vi "Z stage safety.vi"(7 "new position":dbl format="%#_13g", 8 "Error In":errorcluster, 10 "Table Stages":T1={"X Stage"={"Position"=0.0, "Is.Enabled?"=FALSE, "Is.Connected?"=FALSE, "Device SN"="45876539", "AccelerationMaximum"=0.0, "VelocityMaximum"=0.0, "Acceleration"=0.0, "Velocity"=0.0, "waitTimeout (ms)"=0, "Model"=enum."None", "Is.Homed?"=FALSE, "MOVE"=FALSE}, "Y Stage"={"Position"=0.0, "Is.Enabled?"=FALSE, "Is.Connected?"=FALSE, "Device SN"="45876539", "AccelerationMaximum"=0.0, "VelocityMaximum"=0.0, "Acceleration"=0.0, "Velocity"=0.0, "waitTimeout (ms)"=0, "Model"=enum."None", "Is.Homed?"=FALSE, "MOVE"=FALSE}, "Z Stage"={"Position"=0.0, "Is.Enabled?"=FALSE, "Is.Connected?"=FALSE, "Device SN"="45876539", "AccelerationMaximum"=0.0, "VelocityMaximum"=0.0, "Acceleration"=0.0, "Velocity"=0.0, "waitTimeout (ms)"=0, "Model"=enum."None", "Is.Homed?"=FALSE, "MOVE"=FALSE}, "Attenuator"={"Position"=0.0, "Is.Enabled?"=FALSE, "Is.Connected?"=FALSE, "Device SN"="45876539", "AccelerationMaximum"=0.0, "VelocityMaximum"=0.0, "Acceleration"=0.0, "Velocity"=0.0, "waitTimeout (ms)"=0, "Model"=enum."None", "Is.Homed?"=FALSE, "MOVE"=FALSE}}) -> (0 "Error Out":errorcluster, 1 "crash?":bool)   [LabVIEW 2018]
uses:
  Controls/Translation Stage Parameters.ctl
  Hardware Mfg/Thorlabs Translation Stages/Controls/Translation Stage Cluster.ctl
  Controls/Translation Stage Types.ctl
  Controls/Set Get Controls.ctl
  Hardware Mfg/Thorlabs Translation Stages/Controls/Motion Translation Module Control2.ctl
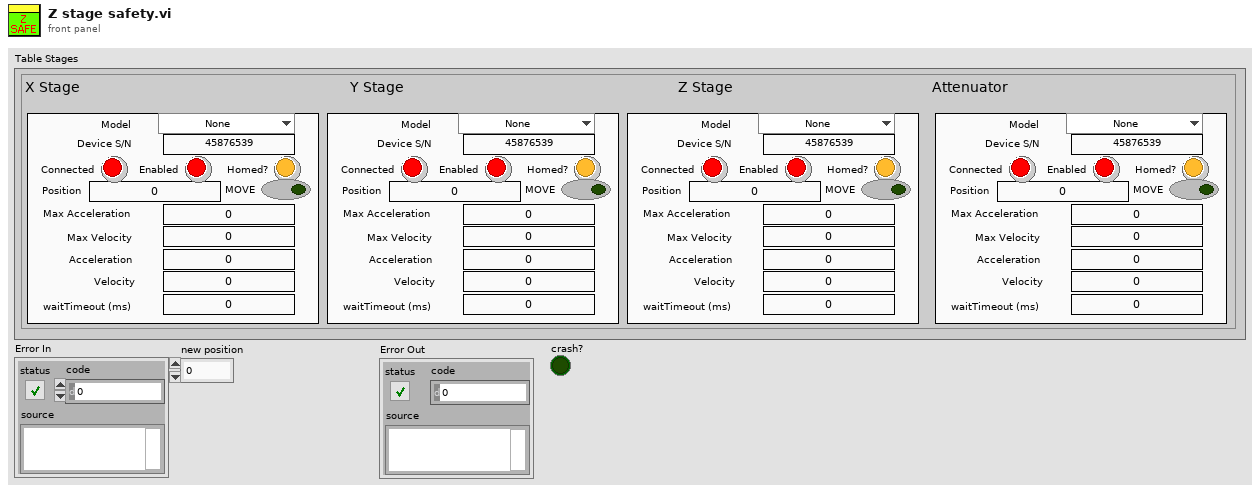
[diagram p1: front panel]
types:
  T1 = typedef "Translation Stage Parameters.ctl" = cluster{"X Stage":T2, "Y Stage":T2, "Z Stage":T2, "Attenuator":T2}
  T2 = typedef "Translation Stage Cluster.ctl" = cluster{"Position":dbl, "Is.Enabled?":bool, "Is.Connected?":bool, "Device SN":string, "AccelerationMaximum":dbl, "VelocityMaximum":dbl, "Acceleration":dbl, "Velocity":dbl, "waitTimeout (ms)":i32, "Model":T3, "Is.Homed?":bool, "MOVE":bool}
  T3 = typedef "Translation Stage Types.ctl" = enum16{"None", "Thorlabs LTS", "Thorlabs MLJ"}
  T4 = typedef "Motion Translation Module Control2.ctl" = enum16{"Init", "Home", "Status", "Velocity/Accel", "Position", "Jog", "Stop", "Uninit", "Enable", "Disable"}
  T5 = typedef "Set Get Controls.ctl" = enum16{"Set", "Get"}
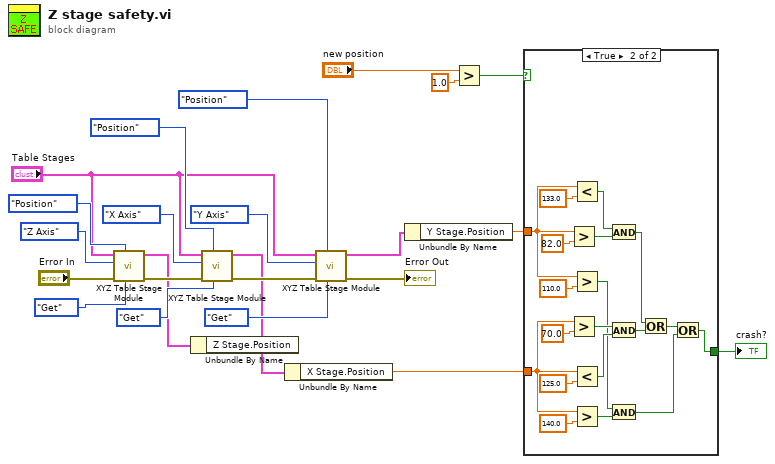
[diagram p0: block diagram]
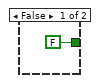
[diagram p2: hidden frame]
diagram:
  n1 = call "XYZ Table Stage Module.vi"("Set/Get"=Set_Get_Controls."Get", "Action"=Motion_Translation_Module_Control2."Position", "Error In"="Error In", "Axis"=enum16{"X Axis", "Y Axis", "Z Axis"}."Z Axis", "Table Stages"="Table Stages") -> ("Error Out"=w16:errorcluster, "Table Stages [out]"=w11:T1)  [unwired: 5 in]
  n2 = Unbundle By Name(w11) -> ()  [unwired: 1 out]
  n3 = call "XYZ Table Stage Module.vi"("Set/Get"=Set_Get_Controls."Get", "Action"=Motion_Translation_Module_Control2."Position", "Error In"=w16, "Axis"=enum16{"X Axis", "Y Axis", "Z Axis"}."X Axis", "Table Stages"="Table Stages") -> ("Error Out"=w12:errorcluster, "Table Stages [out]"=w9:T1)  [unwired: 5 in]
  n4 = Unbundle By Name(w9) -> ("X Stage.Position"=w4:dbl)
  n5 = call "XYZ Table Stage Module.vi"("Set/Get"=Set_Get_Controls."Get", "Action"=Motion_Translation_Module_Control2."Position", "Error In"=w12, "Axis"=enum16{"X Axis", "Y Axis", "Z Axis"}."Y Axis", "Table Stages"="Table Stages") -> ("Error Out"=→"Error Out":errorcluster, "Table Stages [out]"=w10:T1)  [unwired: 5 in]
  n6 = Unbundle By Name(w10) -> ("Y Stage.Position"=w5:dbl)
  n7 = Greater?(x="new position", y=1.0) -> (0:w1:bool)
  n8 = case shown="True" w1 {
    tunnel: [FALSE w25] -> w8
    tunnel: w5 -> [_ w33]
    tunnel: w4 -> [_ w31]
    frame False {
    }
    frame True {
      n9 = Greater?(x=w33, y=82.0) -> (0:w38:bool)
      n10 = Greater?(x=w31, y=70.0) -> (0:w37:bool)
      n11 = Less?(x=w33, y=133.0) -> (x < y?=w39:bool)
      n12 = Greater?(x=w33, y=110.0) -> (0:w29:bool)
      n13 = Less?(x=w31, y=125.0) -> (x < y?=w36:bool)
      n14 = Greater?(x=w31, y=140.0) -> (0:w28:bool)
      n15 = And(x=w39, y=w38) -> (x .and. y?=w34:bool)
      n16 = And(x=w37, y=w36) -> (x .and. y?=w35:bool)
      n17 = And(x=w29, y=w28) -> (x .and. y?=w26:bool)
      n18 = Or(x=w34, y=w35) -> (x .or. y?=w27:bool)
      n19 = Or(x=w27, y=w26) -> (x .or. y?=w25:bool)
    }
  }
  "crash?" <- w8
